vi "VisOpticsErrCodesGenerator.vi"(6 "Error Code base number":i32=9200 min=5000 max=9900, 7 "NHMFL Visible Optics Error Type":T1(ring), 8 "NHMFL Visible Optics Error Categories":T2) -> (0 "user-defined errors Array":errorcluster[](array[cluster]), 1 "Error Code base number output":i32=9200 min=5000 max=9900, 2 "Total user-defined items":u32, 3 "user-defined descriptions":string[](array[string]), 4 "User-defined Error Code":i32, 5 "user-defined codes":i32[](array[numeric]))   [LabVIEW 2019]
doc: "This is to generate user-defined error codes, to be used as Typre-Defs:\nNHMFL Visible Optics Error Categories\nNHMFL Visible Optics Error Type\nNHMFL Visible Optics user-defined error codes\nNHMFL Visible Optics user-defined error descriptions"
uses:
  Globals and TypeDefs/Error Categories.ctt
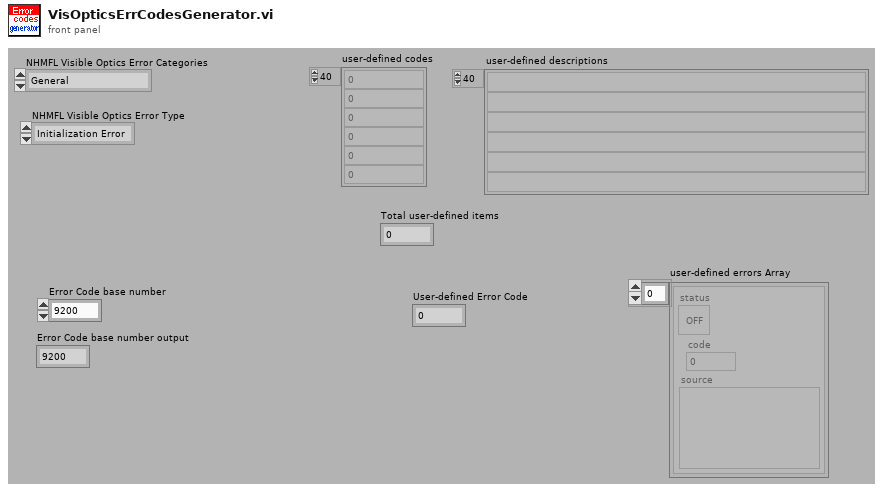
[diagram p1: front panel]
types:
  T1 = enum8{"Initialization Error", "Command Error", "Parameter Error", "Overflow Error", "Time-out Error", "Misc Error", "User cancel"}
  T2 = typedef "Error Categories.ctt" = enum8{"General", "CCD-256x1024", "CCD-1340x400", "InGaAs PDA", "McPherson 2075", "Magnetic Field", "Temperature Control", "Other"}
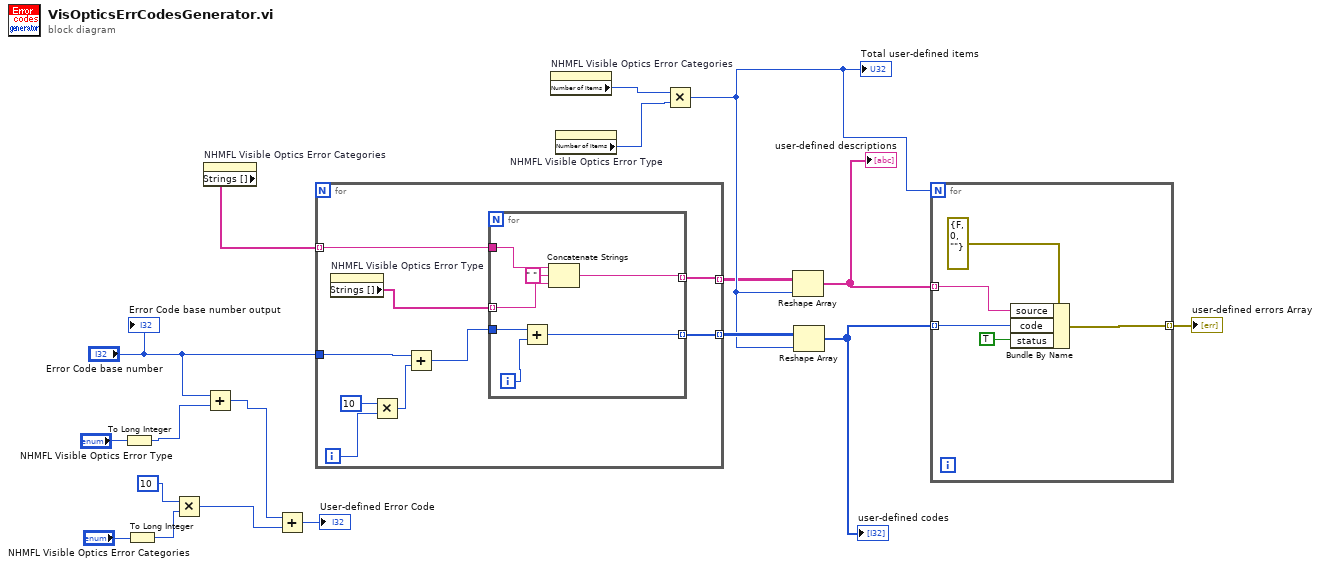
[diagram p0: block diagram]
diagram:
  n1 = To Long Integer(number="NHMFL Visible Optics Error Type") -> (32bit integer=w4:i32)
  n2 = To Long Integer(number="NHMFL Visible Optics Error Categories") -> (32bit integer=w7:i32)
  n3 = Multiply(x=10, y=w7) -> (x*y=w2:i32)
  n4 = property on="NHMFL Visible Optics Error Categories" class="Enum (strict)"() -> ("Strings []"=w18:string[])  [unwired: 2 in, 2 out]
  n5 = Add(x="Error Code base number", y=w4) -> (x+y=w3:i32)
  n6 = Add(x=w3, y=w2) -> (x+y=→"User-defined Error Code":i32)
  n7 = for {
    tunnel: w18 -> [w23] mode=indexing
    tunnel: [w22] -> w10 mode=indexing
    tunnel: [w21] -> w15 mode=indexing
    tunnel: "Error Code base number" -> [w19]
    i -> [w27]
    n8 = property on="NHMFL Visible Optics Error Type" class="Enum (strict)"() -> ("Strings []"=w20:string[])  [unwired: 2 in, 2 out]
    n9 = Multiply(x=10, y=w27) -> (x*y=w25:i32)
    n10 = Add(x=w19, y=w25) -> (x+y=w24:i32)
    n11 = for {
      tunnel: w20 -> [w30] mode=indexing
      tunnel: w24 -> [w33]
      tunnel: [w32] -> w21 mode=indexing
      tunnel: w23 -> [w31]
      tunnel: [w28] -> w22 mode=indexing
      i -> [w34]
      n12 = Add(x=w33, y=w34) -> (x+y=w32:i32)
      n13 = Concatenate Strings(w31, " " ("string"), w30) -> (w28:string)
    }
  }
  n14 = property on="NHMFL Visible Optics Error Categories" class="Enum (strict)"() -> ("Number of Items"=w17:u32)  [unwired: 2 in, 2 out]
  n15 = property on="NHMFL Visible Optics Error Type" class="Enum (strict)"() -> ("Number of Items"=w16:u32)  [unwired: 2 in, 2 out]
  n16 = Multiply(x=w17, y=w16) -> (x*y=w12:u32)
  "Total user-defined items" <- w12
  n17 = Reshape Array(w10, w12) -> (w11:string[])
  "user-defined descriptions" <- w11
  n18 = Reshape Array(w15, w12) -> (w14:i32[])
  "user-defined codes" <- w14
  n19 = for {
    N: w12 -> [_]
    tunnel: w14 -> [w37] mode=indexing
    tunnel: w11 -> [w36] mode=indexing
    tunnel: [w35] -> w13 mode=indexing
    n20 = Bundle By Name(cluster=errorcluster {"status"=FALSE, "code"=0, "source"=""} ("error out"), "source"=w36, "code"=w37, "status"=TRUE) -> (w35:errorcluster)
  }
  "user-defined errors Array" <- w13
  "Error Code base number output" <- "Error Code base number"
